vi "lvstyx_get_dir_length.vi"(2 "error in (no error)":errorcluster, 5 "dir ptr":u32) -> (0 "error out":errorcluster, 1 "dir len":i32)   [LabVIEW 2010, in "lib1299.lvlib"]
uses:
  lib1299.lvlib
  cstyx/win32/cstyx.dll
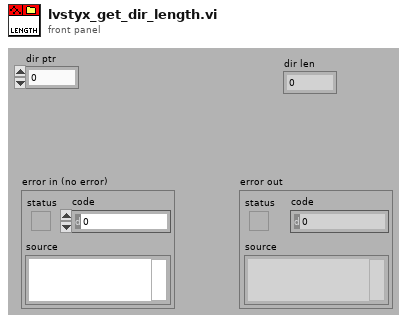
[diagram p1: front panel]
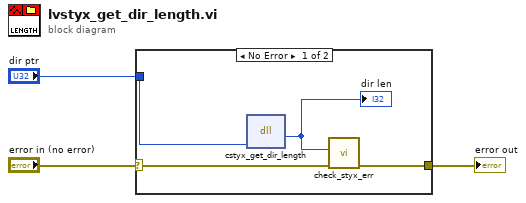
[diagram p0: block diagram]
diagram:
  n1 = case shown="No Error" "error in (no error)" {
    selector: "error in (no error)" -> [w6 w8]
    tunnel: "dir ptr" -> [w7 _]
    tunnel: [w5 w8] -> w2
    frame No Error {
      n2 = dll-call lib="C:/work/ads1299evm/lib_1299/Styx/cstyx/win32/cstyx.dll" fn="cstyx_get_dir_length"("dir"=w7) -> ("len"=w4:i32)  [unwired: 4 in, 2 out]
      "dir len" <- w4
      n3 = call "check_styx_err.vi"("error in (no error)"=w6, "return val"=w4) -> ("error out"=w5:errorcluster)  [unwired: 9 in]
    }
    frame Error {
    }
  }
  "error out" <- w2
